vi "X軸回home_function.vi"(7 "X¶b Home":T1, 8 "error in (no error)":errorcluster) -> (0 "error out":errorcluster)   [LabVIEW 2014]
uses:
  global/Global.vi
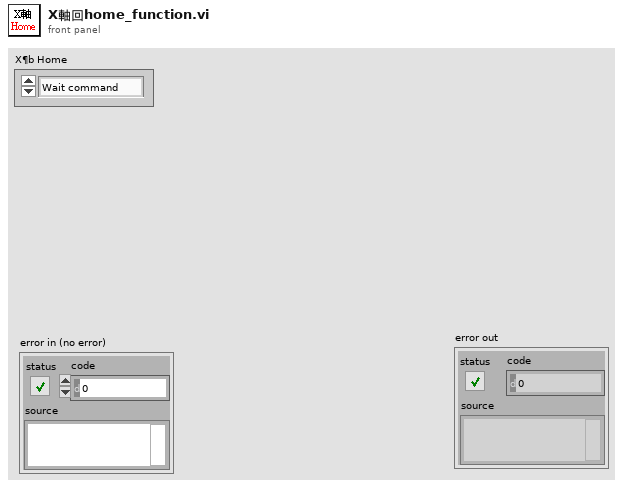
[diagram p1: front panel]
types:
  T1 = typedef "X¶b home_action.ctl" = enum16{"Wait command", "Config X home mode_7", "Start X homing_7", "確認 X homing_7 done", "error"}
  T2 = typedef "軸參數記錄.ctl" = cluster{"X軸取料位":dbl, "X¶bCCD¦ì":dbl, "X軸影像異常排料位":dbl, "X軸迴轉缸位":dbl, "裝完料區已可安全取料位":dbl, "A軸取料角":dbl, "A¶bCCD¨¤":dbl, "B軸取料角":dbl, "B¶bCCD¨¤":dbl, "軸控參數PATH":path, "CCD左連續失敗報警次數":u8, "CCD右連續失敗報警次數":u8, "連續組裝失敗報警次數":u8, "ABVL/VH":i32, "XVL/VH":i32, "AB加速度":i32, "X加速度":i32, "home-XVL/VH":i32, "home-ABVL/VH":i32}
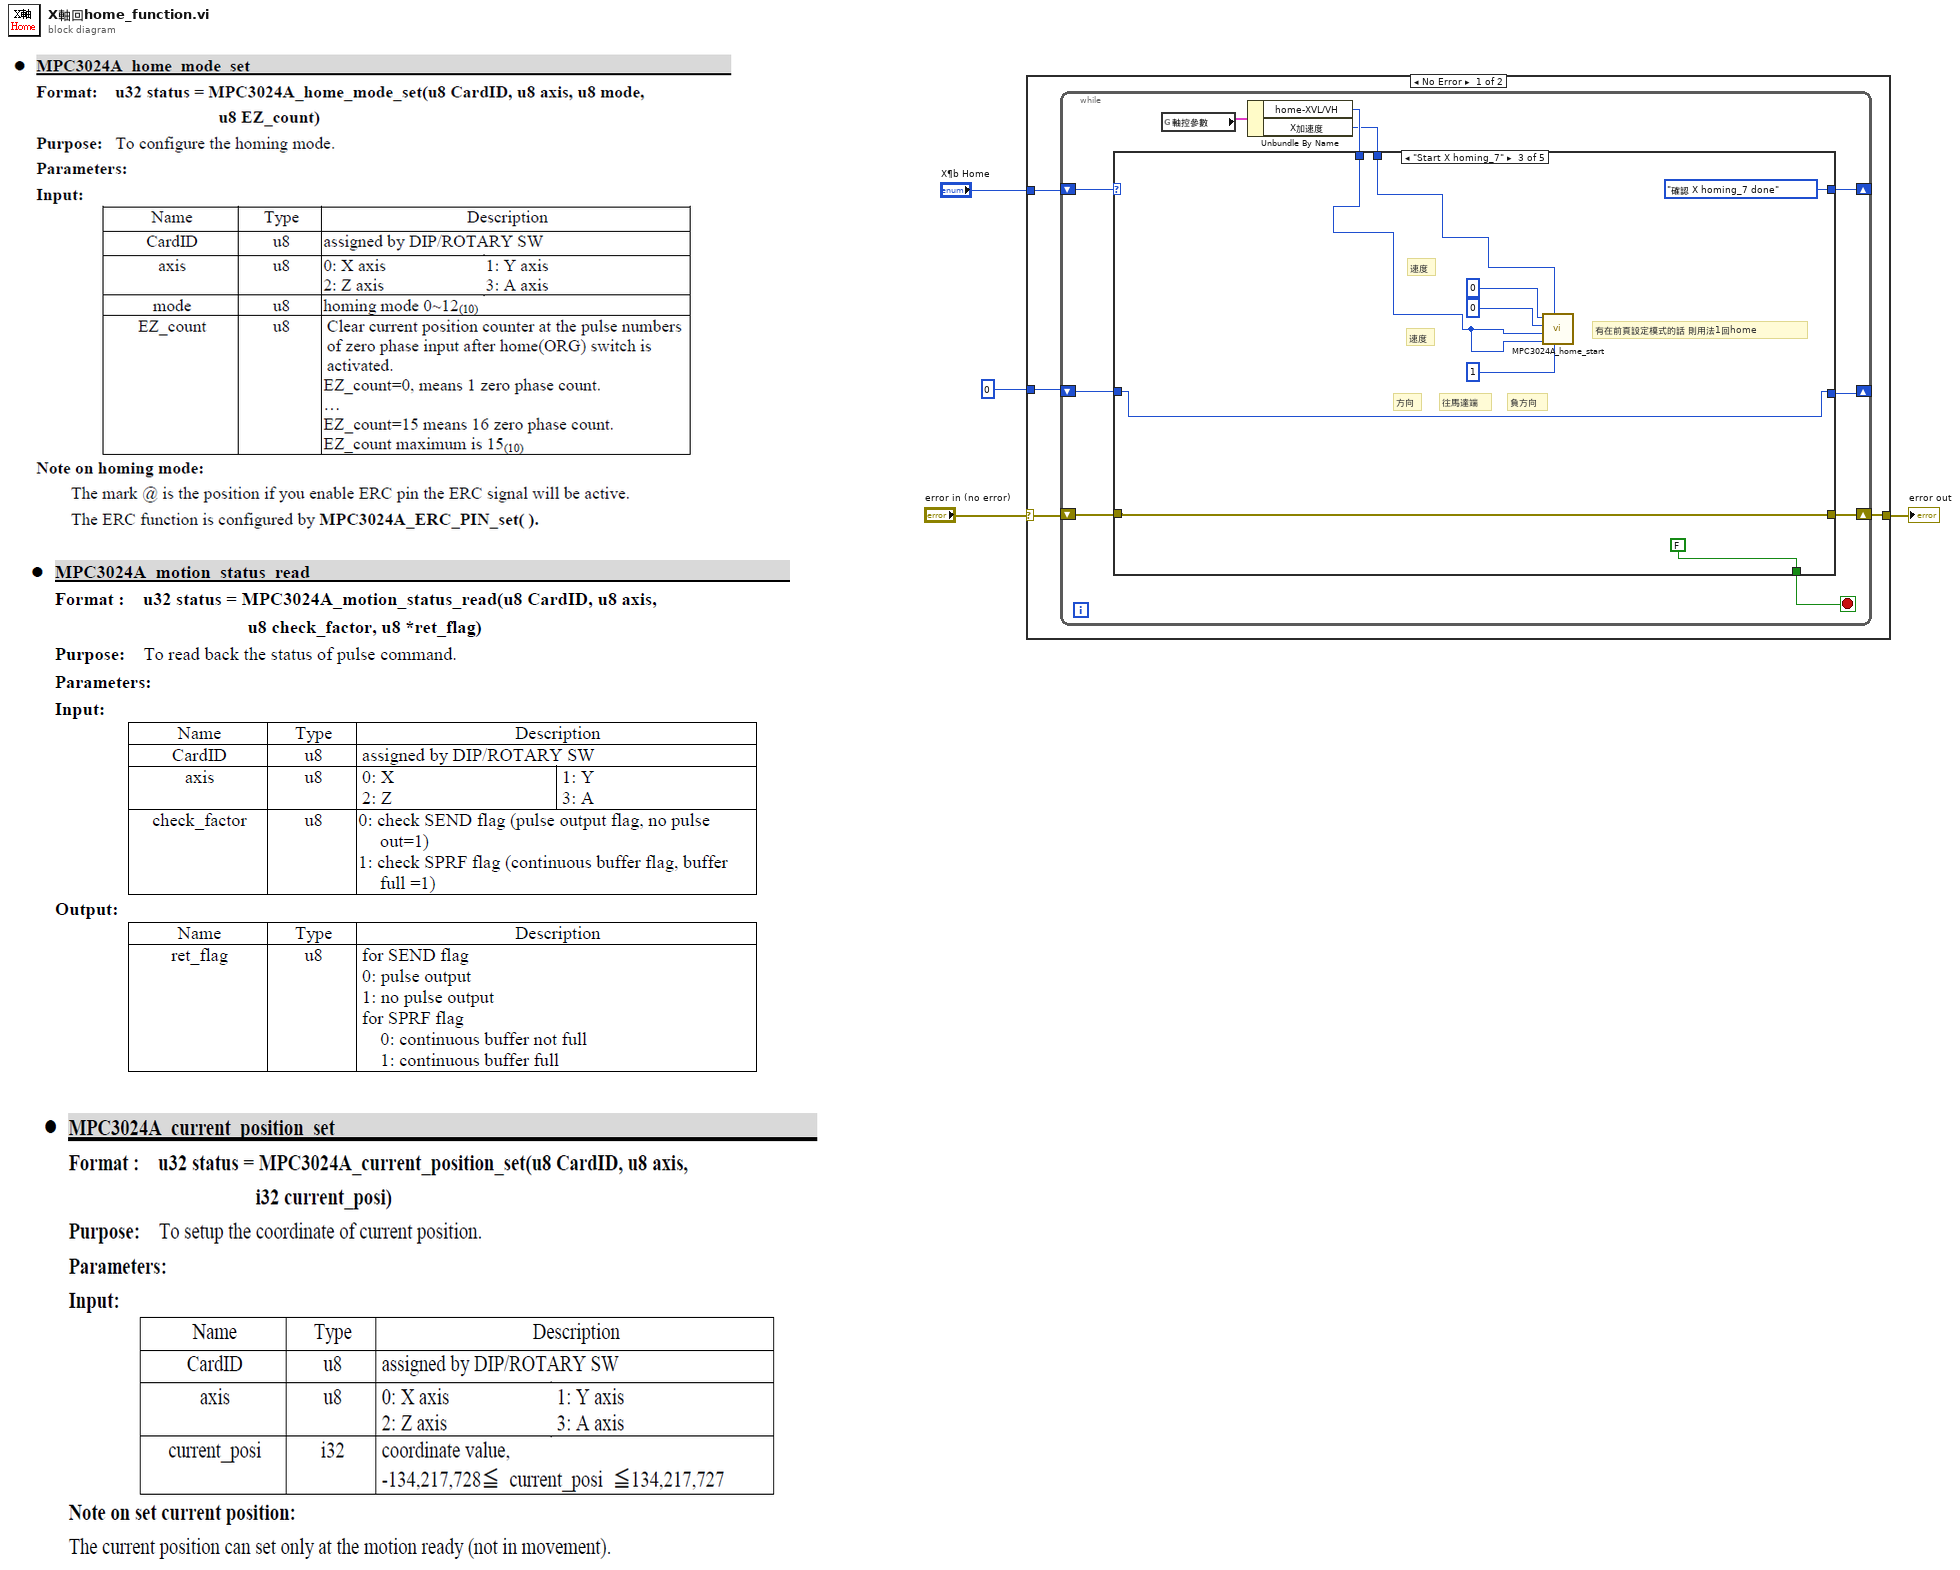
[diagram p0: block diagram]
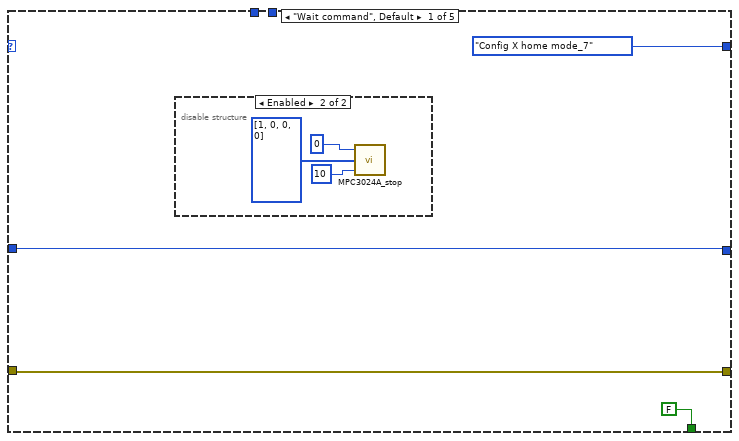
[diagram p2: hidden frame]
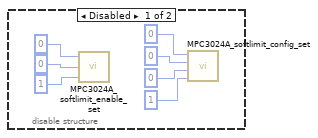
[diagram p3: hidden frame]
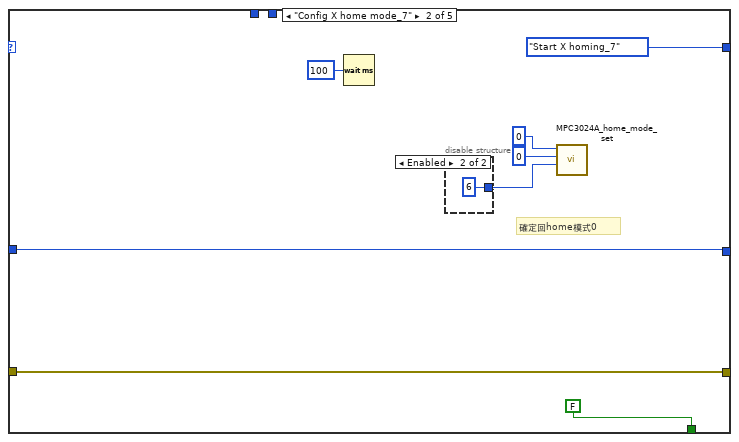
[diagram p4: hidden frame]
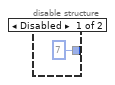
[diagram p5: hidden frame]
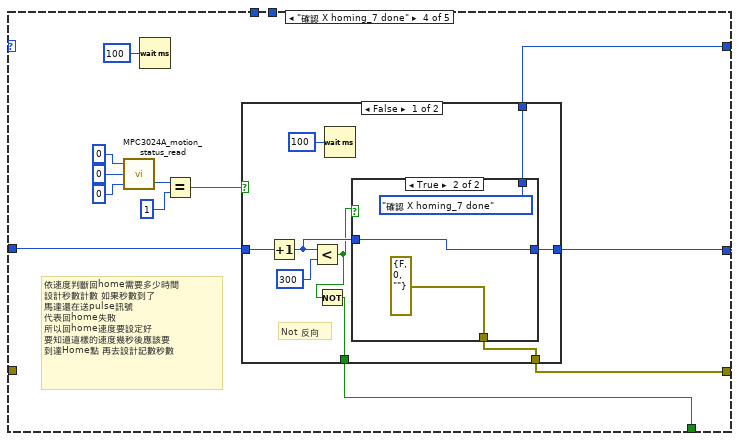
[diagram p6: hidden frame]
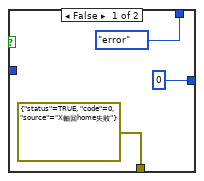
[diagram p7: hidden frame]
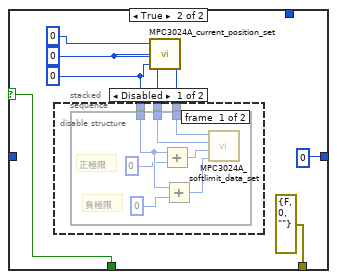
[diagram p8: hidden frame]
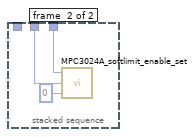
[diagram p9: hidden frame]
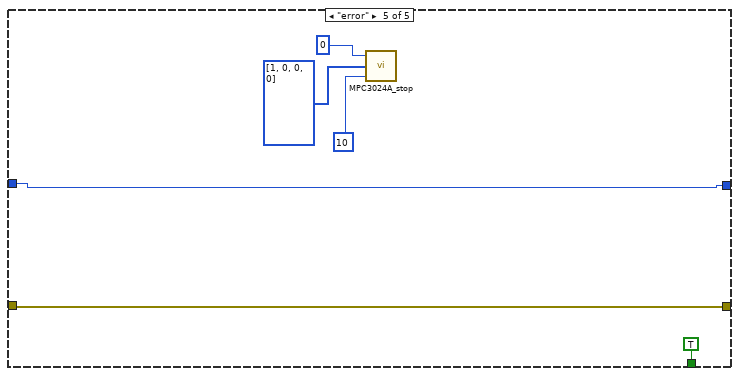
[diagram p11: hidden frame]
diagram:
  n1 = case shown="No Error" "error in (no error)" {
    selector: "error in (no error)" -> [w7 w104]
    tunnel: [w5 w104] -> w3
    tunnel: "X¶b Home" -> [w8 _]
    tunnel: 0 -> [w6 _]
    frame No Error {
      n2 = while {
        shift-right: [w17] -> _
        shift-left: w8 -> [w18]
        shift-right: [w13] -> w5
        shift-left: w7 -> [w12]
        shift-right: [w14] -> _
        shift-left: w6 -> [w15]
        stop <- w16 stop-if-true
        n3 = global read "Global.vi" "軸控參數"() -> (w11:T2)
        n4 = Unbundle By Name(w11) -> ("home-XVL/VH"=w10:i32, "X加速度"=w9:i32)
        n5 = case shown="\"Start X homing_7\"" w18 {
          tunnel: [X¶b_home_action."Config X home mode_7" ("X¶b Home") X¶b_home_action."Start X homing_7" ("X¶b Home") X¶b_home_action."確認 X homing_7 done" ("X¶b Home") w54 _] -> w17
          tunnel: [FALSE FALSE FALSE w53 TRUE] -> w16
          tunnel: w15 -> [w20 w33 w46 w56 w100]
          tunnel: [w20 w33 w46 w55 w100] -> w14
          tunnel: w12 -> [w19 w34 w45 _ w99]
          tunnel: [w19 w34 w45 w52 w99] -> w13
          tunnel: w10 -> [_ _ w44 _ _]
          tunnel: w9 -> [_ _ w43 _ _]
          frame "Wait command", Default {
            n6 = disable-structure shown="Enabled" {
              frame Disabled {
                n7 = call "MPC3024A_softlimit_enable_set.vi"("ON_OFF"=u8 1, "axis"=u8 0, "CardID"=u8 0) -> ()  [unwired: 1 out]
                n8 = call "MPC3024A_softlimit_config_set.vi"("SL_action"=u8 1, "source_sel"=u8 0, "axis"=u8 0, "CardID"=u8 0) -> ()  [unwired: 1 out]
              }
              frame Enabled {
                n9 = call "MPC3024A_stop.vi"("Tdec_ms"=u32 10, "axis[4]"=u8[] [1, 0, 0, 0], "CardID"=u8 0) -> ()  [unwired: 1 out]
              }
            }
          }
          frame "Config X home mode_7" {
            # "確定回home模式0"
            n10 = Wait (ms)(milliseconds to wait=u32 100) -> ()  [unwired: 1 out]
            n11 = disable-structure shown="Enabled" {
              disable-tunnel: [u8 7 ("mode") u8 6 ("mode")] -> w39
              frame Disabled {
              }
              frame Enabled {
              }
            }
            n12 = call "MPC3024A_home_mode_set.vi"("mode"=w39, "axis"=u8 0, "CardID"=u8 0) -> ()  [unwired: 1 in, 1 out]
          }
          frame "Start X homing_7" {
            # "負方向"
            # "往馬達端"
            # "有在前頁設定模式的話 則用法1回home"
            # "速度"
            # "速度"
            # "方向"
            n13 = call "MPC3024A_home_start.vi"("direction"=u8 1, "Tacc_ms"=w43, "VH"=w44, "VL"=w44, "axis"=u8 0, "CardID"=u8 0) -> ()  [unwired: 1 out]
          }
          frame "確認 X homing_7 done" {
            # "依速度判斷回home需要多少時間\n設計秒數計數 如果秒數到了\n馬達還在送pulse訊號\n代表回home失敗\n所以回home速度要設定好 \n要知道這樣的速度幾秒後應該要\n到達Home點 再去設計記數秒數"
            n14 = call "MPC3024A_motion_status_read.vi"("check_factor"=u8 0, "axis"=u8 0, "CardID"=u8 0) -> ("ret_fig"=w62:u8)  [unwired: 1 out]
            n15 = Wait (ms)(milliseconds to wait=u32 100) -> ()  [unwired: 1 out]
            n16 = Equal?(x=w62, y=u8 1) -> (x = y?=w57:bool)
            n17 = case shown="False" w57 {
              selector: w57 -> [_ w82]
              tunnel: [w70 errorcluster {"status"=FALSE, "code"=0, "source"=""} ("error in (no error)")] -> w52
              tunnel: [w71 0] -> w55
              tunnel: w56 -> [w69 _]
              tunnel: [w64 w82] -> w53
              tunnel: [w67 _] -> w54
              frame False {
                # "Not 反向"
                n18 = Increment(x=w69) -> (x+1=w72:i32)
                n19 = Less?(x=w72, y=300) -> (x < y?=w65:bool)
                n20 = Not(x=w65) -> (.not. x?=w64:bool)
                n21 = Wait (ms)(milliseconds to wait=u32 100) -> ()  [unwired: 1 out]
                n22 = case shown="True" w65 {
                  tunnel: [0 w77] -> w71
                  tunnel: w72 -> [_ w77]
                  tunnel: [errorcluster {"status"=TRUE, "code"=0, "source"="X軸回home失敗"} ("error in (no error)") errorcluster {"status"=FALSE, "code"=0, "source"=""} ("error in (no error)")] -> w70
                  tunnel: [X¶b_home_action."error" ("X¶b Home") X¶b_home_action."確認 X homing_7 done" ("X¶b Home")] -> w67
                  frame False {
                  }
                  frame True {
                  }
                }
              }
              frame True {
                w81 = u8 0 ("value")
                w80 = u8 0 ("value")
                w79 = 0 ("value")
                n23 = disable-structure shown="Disabled" {
                  disable-tunnel: w81 -> [w87 _]
                  disable-tunnel: w80 -> [w86 _]
                  disable-tunnel: w79 -> [w85 _]
                  frame Disabled {
                    n24 = stacked-sequence {
                      tunnel: w87 -> [w94 w97]
                      tunnel: w86 -> [w93 w96]
                      tunnel: w85 -> [w92 _]
                      frame #0 {
                        # "負極限"
                        # "正極限"
                        n25 = Add(x=w92, y=0) -> (x+y=w91:i32)
                        n26 = Add(x=w92, y=0) -> (x+y=w90:i32)
                        n27 = call "MPC3024A_softlimit_data_set.vi"("N_limit"=w90, "P_limit"=w91, "axis"=w93, "CardID"=w94) -> ()  [unwired: 1 out]
                      }
                      frame #1 {
                        n28 = call "MPC3024A_softlimit_enable_set.vi"("ON_OFF"=u8 0, "axis"=w96, "CardID"=w97) -> ()  [unwired: 1 out]
                      }
                    }
                  }
                  frame Enabled {
                  }
                }
                n29 = call "MPC3024A_current_position_set.vi"("current_posi"=w79, "axis"=w80, "CardID"=w81) -> ()  [unwired: 1 out]
              }
            }
          }
          frame "error" {
            n30 = call "MPC3024A_stop.vi"("Tdec_ms"=u32 10, "axis[4]"=u8[] [1, 0, 0, 0], "CardID"=u8 0) -> ()  [unwired: 1 out]
          }
        }
      }
    }
    frame Error {
    }
  }
  "error out" <- w3
